vi "GetRefrigSystemStatus.vi"(0 "VISA resource name":refnum<visa-resource-name>, 5 "Refrigeration system number (1-4)":T1=1 items=["Channel 1"=1, "Channel 2"=2, "Channel 3"=3, "Channel 4"=4], 11 "error in":errorcluster) -> (4 "VISA resource name out":refnum<visa-resource-name>, 6 "Refrigeration system status string":string, 8 "Refrigeration system status":i32, 10 "Refrigeration system status binary string":string, 15 "error out":errorcluster)   [LabVIEW 2023, in "Thermotron 8800.lvlib"]
doc: "RDAT\nCommand name: Send refrigeration system status\nCommand type: System status\nDescription: This command returns a binary-coded decimal value that displays the status for the refrigeration data. The bits for each data group are explained below:\nSyntax: RDATn?\nWhere:\nn = the refrigeration system number (1 through 4)\nBits Meaning \n0 and 1 Transducer #4 status \n2 and 3 Transducer #3 status \n4 and 5 Transducer #2 status\n6 and 7 Transducer #1 status \n8 through 11 Highstage compressor status \n12 through 15 Low-stage compressor status\n16 and 17 Refrig. temperature status\nTransducer #1 Transducer #2 Transducer #3\nbit 7 bit 6 bit 5 bit 4 bit 3 bit 2 \nTransducer #4\nbit 1 bit 0\nRefrig. temp. Low-stage compressor\nbit 17 bit 16 bit 15 bit 14 bit 13 bit 12 \nHigh-stage compressor\nbit 11 bit 10 bit 9 bit 8\nFor transducer and refrig. temperature status values:\n00 = okay 01 = trip 10 = trip delay\nFor high-stage and low-stage compressor status values:\n0000 = off 0001 = on 0010 = pump-down 0011 = tripped 0100 = on delay\nData type: Coded integer\nQuery example 1: RDAT2?\n8800 response: 832 = 0000000011 01000000\nTransducer #1 Transducer #2 Transducer #3\nbit 7: 0 bit 6: 1 bit 5: 0 bit 4: 0 bit 3: 0 bit 2:0 \nTransducer #4\nbit 1: 0 bit 0: 0\nRefrig. temp. Low-stage compressor\nbit 17:0 bit 16:0 bit 15:0 bit 14:0 bit 13:0 bit 12:0 \nHigh-stage compressor\nbit 11: 0 bit 10: 0 bit 9: 1 bit 8: 1\n(Transducer #1 has tripped and the high-stage compressor has tripped.)\nQuery example 2: RDAT1?\n8800 response: 0 (Transducers 1 through 4 are okay, the high-stage and low-stage compressors are off, and the refrig. temperature is okay.)"
uses:
  Thermotron 8800.lvlib
  Private/AnalogInputChannelNumber 1-4.ctl
panel:
  out "concatenated string":string
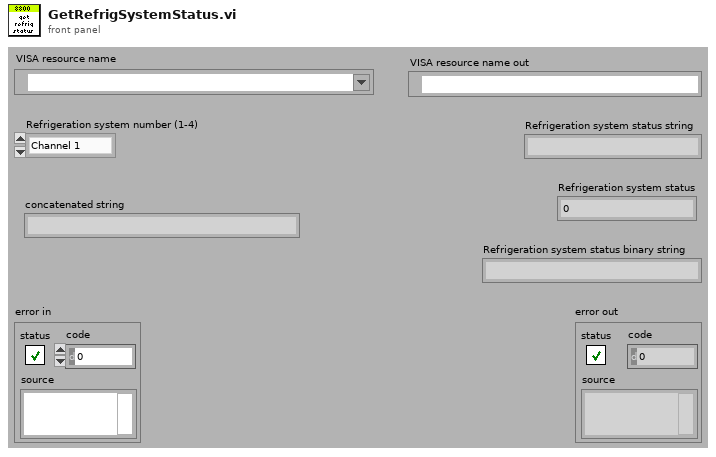
[diagram p1: front panel]
types:
  T1 = typedef "Thermotron 8800.lvlib/AnalogInputChannelNumber 1-4.ctl" = u16
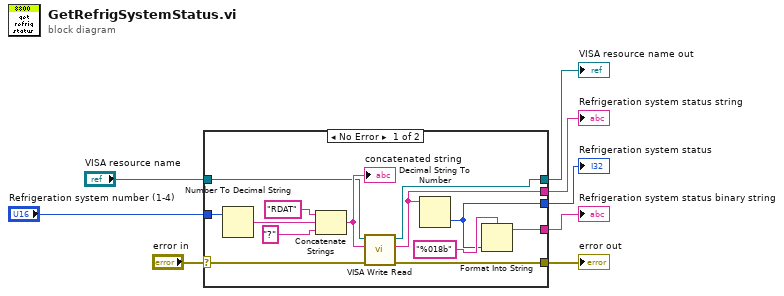
[diagram p0: block diagram]
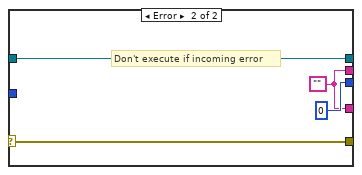
[diagram p2: hidden frame]
diagram:
  n1 = case shown="No Error" "error in" {
    selector: "error in" -> [w19 w25]
    tunnel: [w18 w25] -> w7
    tunnel: "VISA resource name" -> [w17 w24]
    tunnel: [w16 w24] -> w5
    tunnel: [w15 w22] -> w4
    tunnel: [w9 0] -> w3
    tunnel: "Refrigeration system number (1-4)" -> [w13 _]
    tunnel: [w11 w22] -> w1
    frame No Error {
      n2 = Number To Decimal String(number=w13) -> (decimal integer string=w12:string)  [unwired: 1 in]
      n3 = Concatenate Strings("RDAT" ("8800 Command"), w12, "?" ("8800 Command")) -> (w20:string)
      "concatenated string" <- w20
      n4 = call "VISA Write Read.vi"("error in (no error)"=w19, "8800 Command"=w20, "VISA Refnum in"=w17) -> ("error out"=w18:errorcluster, "read buffer"=w15:string, "VISA Refnum out"=w16:refnum<visa-resource-name>)  [unwired: 6 in]
      n5 = Decimal String To Number(string=w15) -> (number=w9:i32)  [unwired: 2 in, 1 out]
      n6 = Format Into String(format string="%018b", w9) -> (resulting string=w11:string)  [unwired: 2 in, 1 out]
    }
    frame Error {
      w22 = ""
      # "Don't execute if incoming error"
    }
  }
  "error out" <- w7
  "VISA resource name out" <- w5
  "Refrigeration system status string" <- w4
  "Refrigeration system status" <- w3
  "Refrigeration system status binary string" <- w1
